vi "Add Animation.vi"(8 "Error In":errorcluster, 10 "Animation":refnum<class "Animation.lvclass">, 11 "Display Manager In":refnum<class "Display Manager.lvclass">) -> (0 "Error Out":errorcluster, 3 "Display Manager Out":refnum<class "Display Manager.lvclass">)   [LabVIEW 2021, in "Display Manager.lvclass"]
uses:
  Display Manager.lvclass
  Display Manager.lvclass/Display Manager.ctl
  Animation/Animation.lvclass
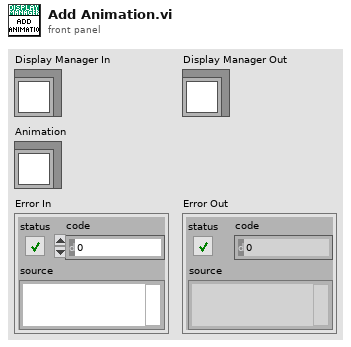
[diagram p1: front panel]
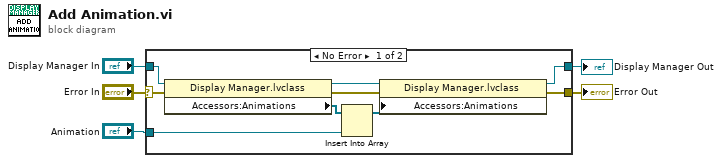
[diagram p0: block diagram]
diagram:
  n1 = case shown="No Error" "Error In" {
    selector: "Error In" -> [w13 w15]
    tunnel: "Display Manager In" -> [w14 w16]
    tunnel: [w10 w16] -> w3
    tunnel: [w11 w15] -> w2
    tunnel: "Animation" -> [w7 _]
    frame No Error {
      n2 = property class="Display Manager.lvclass"(reference=w14, error in=w13) -> (reference out=w12:refnum<class "Display Manager.lvclass">, error out=w8:errorcluster, "Accessors:Animations"=w9:refnum<class "Animation.lvclass">[])
      n3 = Insert Into Array(array=w9, new element=w7) -> (w6:refnum<class "Animation.lvclass">[])  [unwired: 1 in]
      n4 = property class="Display Manager.lvclass"(reference=w12, error in=w8, "Accessors:Animations"=w6) -> (reference out=w10:refnum<class "Display Manager.lvclass">, error out=w11:errorcluster)
    }
    frame Error {
    }
  }
  "Display Manager Out" <- w3
  "Error Out" <- w2
